vi "Get Element TD from Array TD.vi"(8 "error in (no error)":errorcluster, 10 "Array Type Descriptor":refnum<class "Array.lvclass">) -> (0 "error out":errorcluster, 2 "Element Type Descriptor":refnum<class "TD.lvclass">)   [LabVIEW 2020, in "variant.lvlib" / "type.lvlib" / "Array.lvclass"]
doc: "Returns the type descriptor of the array element."
uses:
  Array.lvclass
  TD.lvclass
  C:/projects/OpenG-Variant-Data-Library/source/library/Bytes/Bytes.lvclass
  C:/projects/OpenG-Variant-Data-Library/source/library/LVData/Type Descriptor/TD.lvclass
  Bytes/Bytes.lvclass/Bytes.ctl
  c017a9a8-ccc5-4ad4-8ab9-cbac41437c25.vi
  get_num_elements.vi/b3898c1b-5169-4cb1-894b-457c92b4a1c3.vi
  c017a9a8-ccc5-4ad4-8ab9-cbac41437c25.vi/81433c74-ee36-47cf-a886-10c868675b30.vi
  c017a9a8-ccc5-4ad4-8ab9-cbac41437c25.vi/d8d9ff34-2c15-4edb-a5ad-7260f11560db.vi
  Bytes/from_byte_array.vi
  get_num_elements.vi/b3898c1b-5169-4cb1-894b-457c92b4a1c3.vi/81433c74-ee36-47cf-a886-10c868675b30.vi
  get_num_elements.vi/b3898c1b-5169-4cb1-894b-457c92b4a1c3.vi/d8d9ff34-2c15-4edb-a5ad-7260f11560db.vi
  Bytes/to_data.vi
  Bytes/Bytes.lvclass
panel:
  # "[OpenG VI Tags] ***Do Not Remove***"
  # "Get Array Element TD.vi\n\nReturns the type descriptor of the array element.\n\nPlease visit http://www.OpenG.org to learn about the\nOpen Source LabVIEW software movement.\n\nNOTICE -- YOU MUST LEAVE THIS NOTICE IN PLACE.  PER THE TERMS OF THE LICENSE BELOW, YOU MAY SUBLICENSE THIS SOFTWARE \nIN ANY WAY THAT DOES NOT CONFLICT WITH THIS LICENSE.\n\n### BSD License (http://www.opensource.org/licenses/bsd-license.php) Begin ###\n \nCopyright (c) 2002, Jean-Pierre Drolet <drolet_jp@hotmail.com>\nCopyright (c) 2002-2006, Jim Kring <jim@jimkring.com>\n\nAll rights reserved.\n\nRedistribution and use in source and binary forms, with or without modification, are permitted provided that the following conditions are met:\n\n    * Redistributions of source code must retain the above copyright notice, this list of conditions and the following disclaimer.\n    * Redistributions in binary form must reproduce the above copyright notice, this list of conditions and the following disclaimer in the \n       documentation and/or other materials provided with the distribution.\n    * Neither the name of SciWare, James Kring, Inc., nor the names of its contributors may be used to endorse or promote products derived \n       from this software without specific prior written permission.\n\nTHIS SOFTWARE IS PROVIDED BY THE COPYRIGHT HOLDERS AND CONTRIBUTORS \"AS IS\" AND ANY EXPRESS OR IMPLIED WARRANTIES, \nINCLUDING, BUT NOT LIMITED TO, THE IMPLIED WARRANTIES OF MERCHANTABILITY AND FITNESS FOR A PARTICULAR PURPOSE ARE \nDISCLAIMED. IN NO EVENT SHALL THE COPYRIGHT OWNER OR CONTRIBUTORS BE LIABLE FOR ANY DIRECT, INDIRECT, INCIDENTAL,\n SPECIAL, EXEMPLARY, OR CONSEQUENTIAL DAMAGES (INCLUDING, BUT NOT LIMITED TO, PROCUREMENT OF SUBSTITUTE GOODS OR \nSERVICES; LOSS OF USE, DATA, OR PROFITS; OR BUSINESS INTERRUPTION) HOWEVER CAUSED AND ON ANY THEORY OF LIABILITY, \nWHETHER IN CONTRACT, STRICT LIABILITY, OR TORT (INCLUDING NEGLIGENCE OR OTHERWISE) ARISING IN ANY WAY OUT OF THE USE \nOF THIS SOFTWARE, EVEN IF ADVISED OF THE POSSIBILITY OF SUCH DAMAGE.\n\n### BSD License End ###"
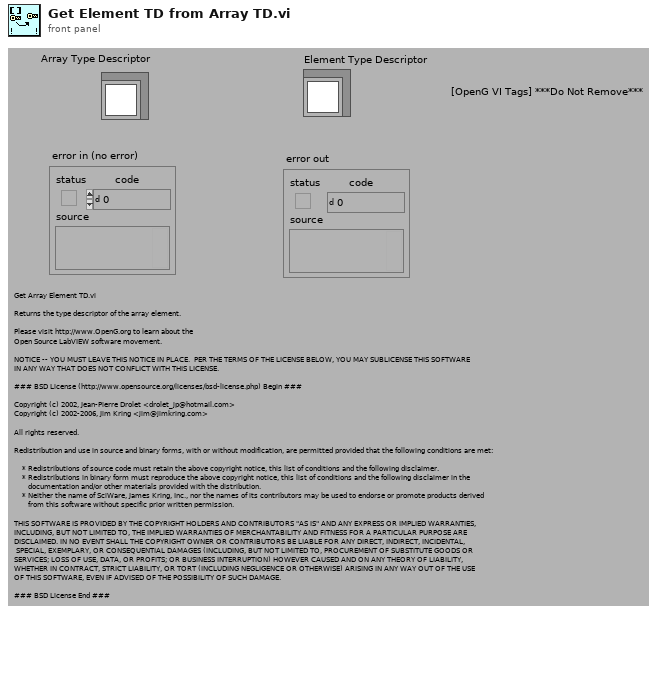
[diagram p1: front panel]
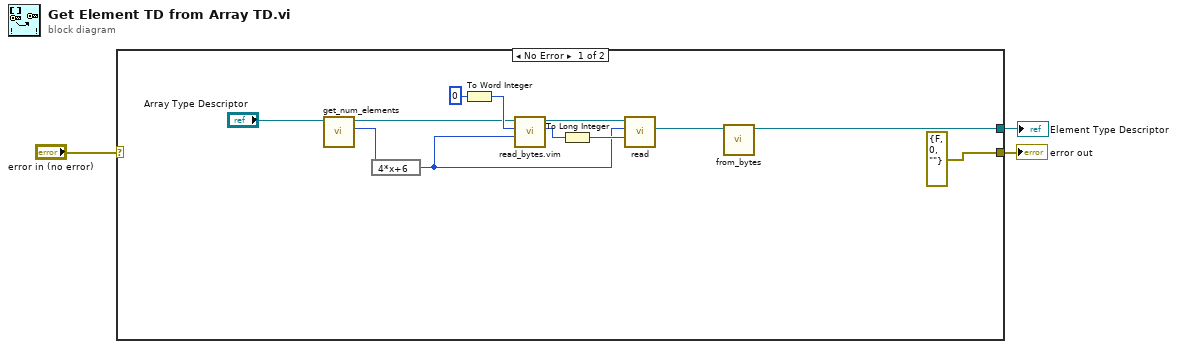
[diagram p0: block diagram]
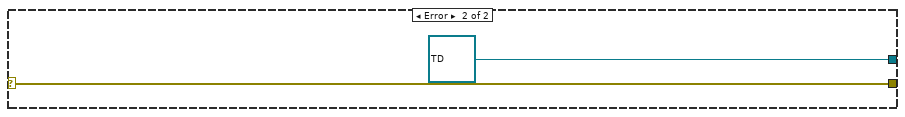
[diagram p2: hidden frame]
diagram:
  n1 = case shown="No Error" "error in (no error)" {
    selector: "error in (no error)" -> [_ w17]
    tunnel: [errorcluster {"status"=FALSE, "code"=0, "source"=""} ("error out") w17] -> w3
    tunnel: [w4 refnum<class "TD.lvclass"> refnum ("TypeDescriptor")] -> w1
    frame No Error {
      n2 = call "get_num_elements.vi"("TypeDescriptor"="Array Type Descriptor") -> ("num_element"=w13:i32, "TypeDescriptor out"=w10:refnum<class "Array.lvclass">)  [unwired: 9 in]
      n3 = expression code="4*x+6"(w13) -> (w6:i32)
      n4 = To Word Integer(number=0) -> (16bit integer=w11:i16)
      n5 = call "read_bytes.vim"("byte offset"=w6, "data type"=w11, "Bytes in"=w10) -> ("value"=w8:i16, "Bytes out"=w9:refnum<class "Array.lvclass">)  [unwired: 7 in]
      n6 = To Long Integer(number=w8) -> (32bit integer=w7:i32)
      n7 = call "read.vi"("length (-1: rest)"=w7, "offset (-1: current position)"=w6, "Bytes in"=w9) -> ("Bytes read"=w5:refnum<class "Bytes.lvclass">)  [unwired: 7 in, 1 out]
      n8 = call "from_bytes.vi"("Bytes"=w5) -> ("TypeDescriptor"=w4:refnum<class "TD.lvclass">)  [unwired: 10 in]
    }
    frame Error {
    }
  }
  "error out" <- w3
  "Element Type Descriptor" <- w1
